vi "set_WL_WN_mode.vi"(8 "error in":errorcluster, 10 "Measure Type":enum16{"Wavelength", "Wavenumber"}(ring), 11 "address":string) -> (0 "error out":errorcluster)   [LabVIEW 2020]
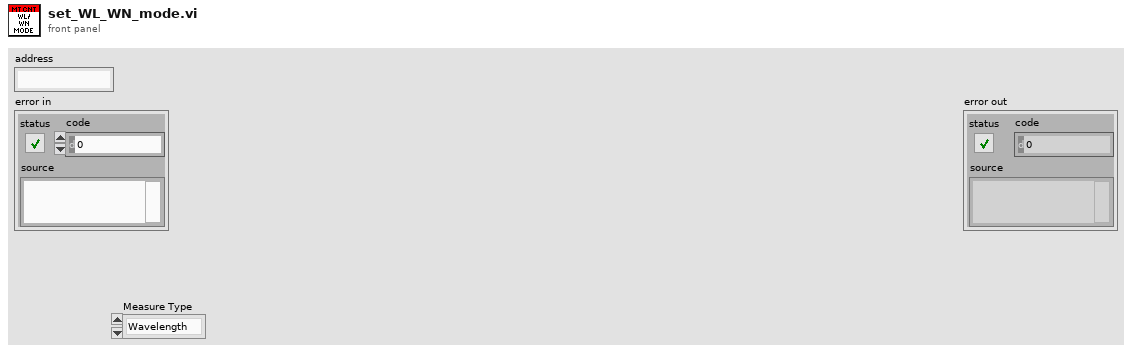
[diagram p1: front panel]
types:
  T1 = enum16{"Standard", "Buffered", "CRLF", "Immediate"}
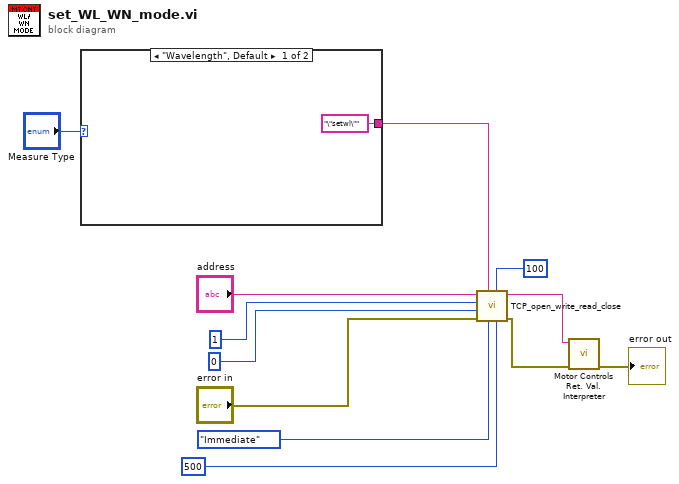
[diagram p0: block diagram]
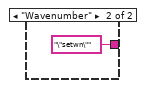
[diagram p2: hidden frame]
diagram:
  n1 = case shown="\"Wavelength\", Default" "Measure Type" {
    tunnel: ["\"setwl\"" "\"setwn\""] -> w1
    frame "Wavelength", Default {
    }
    frame "Wavenumber" {
    }
  }
  n2 = call "TCP_open_write_read_close.vi"("timeout ms (25000)"=500, "bytes to read"=100, "mode (standard)"=T1."Immediate", "write string"=w1, "error in"="error in", "local port (0)"=u16 0, "remote port or service name"=u16 1, "address"="address") -> ("error out"=w6:errorcluster, "read string"=w4:string)  [unwired: 2 in]
  n3 = call "Motor Controls Ret. Val. Interpreter.vi"("error in"=w6, "Command Return"=w4) -> ("error out"=→"error out":errorcluster)  [unwired: 8 in, 1 out]
